vi "DAQNavi Read (Analog 1D DBL 1Chan NSamp).vi"(8 "error in (no error)":errorcluster, 9 "number of samples per channel to read":u32=1000, 10 "timeout":dbl=10.0, 11 "task in":i32) -> (0 "error out":errorcluster, 1 "markBuf":cluster{"Data Index":i64, "SrcId":i64}[](array[cluster]), 2 "data":dbl[](array[numeric]), 3 "task out":i32)   [LabVIEW 2020]
uses:
  DAQNavi_LV.dll
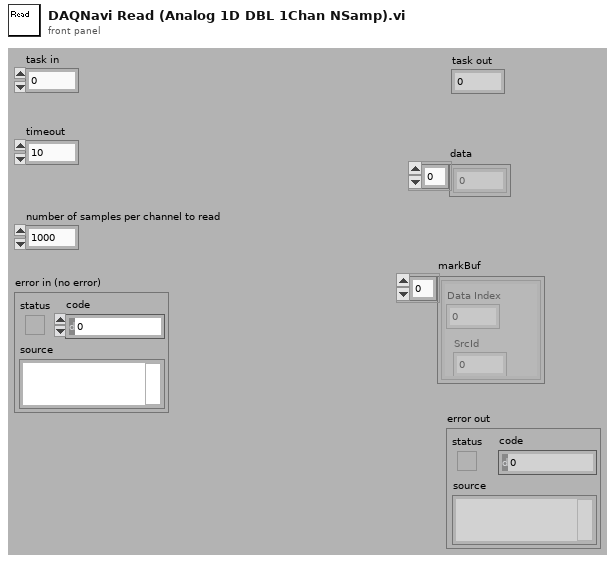
[diagram p1: front panel]
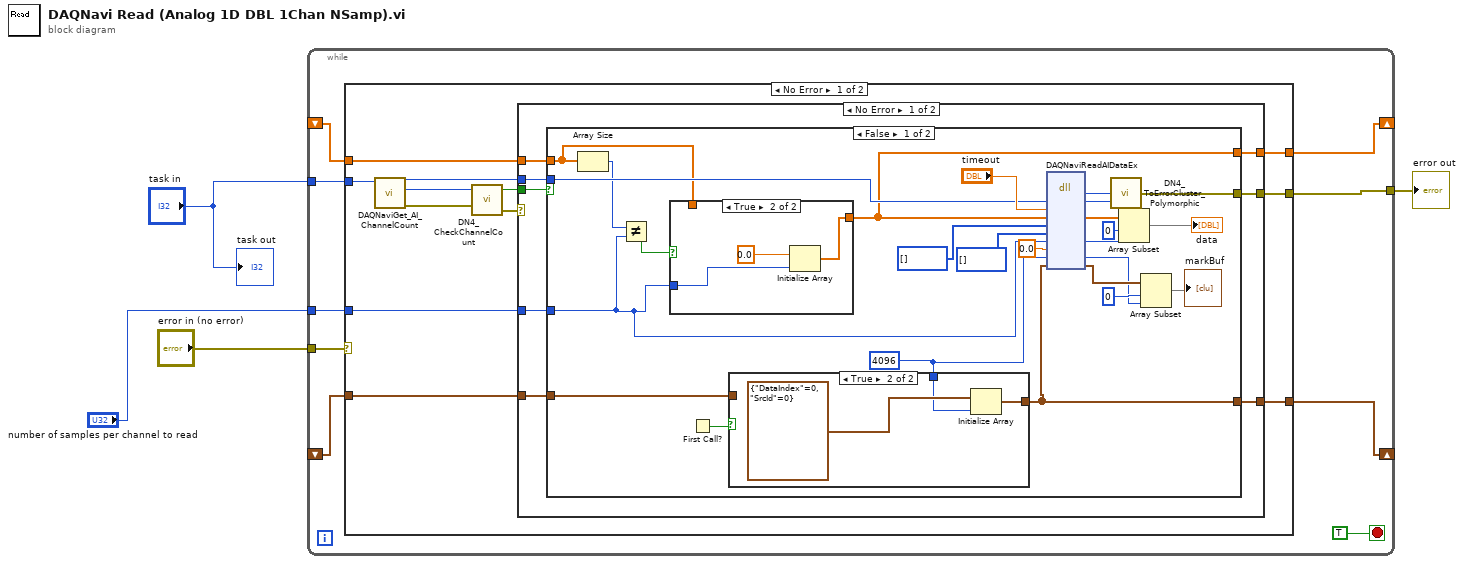
[diagram p0: block diagram]
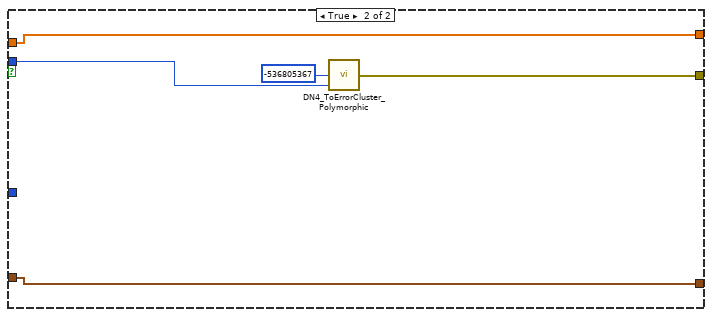
[diagram p4: hidden frame]
diagram:
  n1 = while {
    tunnel: "error in (no error)" -> [w13]
    tunnel: [w12] -> w3
    tunnel: "task in" -> [w11]
    tunnel: "number of samples per channel to read" -> [w10]
    shift-right: [w8] -> _
    shift-left: _ -> [w7]
    shift-right: [w6] -> _
    shift-left: _ -> [w5]
    stop <- TRUE stop-if-true
    n2 = case shown="No Error" w13 {
      selector: w13 -> [_ w77]
      tunnel: w11 -> [w24 _]
      tunnel: [w25 w77] -> w12
      tunnel: w10 -> [w18 _]
      tunnel: [w17 w76] -> w8
      tunnel: w7 -> [w16 w76]
      tunnel: [w15 w75] -> w6
      tunnel: w5 -> [w14 w75]
      frame No Error {
        n3 = call "DAQNaviGet_AI_ChannelCount.vi"("task in"=w24) -> ("error out"=w22:errorcluster, "channel count"=w23:i32, "task out"=w19:i32)  [unwired: 1 in, 7 out]
        n4 = call "DN4_CheckChannelCount.vi"("error out"=w22, "channel count"=w23) -> ("error IO"=w20:errorcluster, "greater than 1?"=w21:bool)  [unwired: 2 out]
        n5 = case shown="No Error" w20 {
          selector: w20 -> [_ w74]
          tunnel: w21 -> [w33 _]
          tunnel: [w32 w74] -> w25
          tunnel: w19 -> [w31 _]
          tunnel: w18 -> [w30 _]
          tunnel: [w29 w73] -> w17
          tunnel: w16 -> [w28 w73]
          tunnel: [w27 w72] -> w15
          tunnel: w14 -> [w26 w72]
          frame No Error {
            n6 = case shown="False" w33 {
              tunnel: [w54 w70] -> w32
              tunnel: w31 -> [w53 w69]
              tunnel: w30 -> [w43 _]
              tunnel: [w45 w68] -> w29
              tunnel: w28 -> [w44 w68]
              tunnel: [w38 w67] -> w27
              tunnel: w26 -> [w40 w67]
              frame False {
                w39 = 4096 ("startTime")
                n7 = Array Size(array=w44) -> (size(s)=w47:i32)
                n8 = Not Equal?(x=w47, y=w43) -> (x != y?=w46:bool)
                n9 = case shown="True" w46 {
                  tunnel: w43 -> [_ w65]
                  tunnel: [w63 w64] -> w45
                  tunnel: w44 -> [w63 _]
                  frame False {
                  }
                  frame True {
                    n10 = Initialize Array(0.0 ("element"), w65) -> (w64:dbl[])
                  }
                }
                n11 = First Call?() -> (First Call?: T/F=w41:bool)
                n12 = case shown="True" w41 {
                  tunnel: w39 -> [_ w61]
                  tunnel: [w59 w60] -> w38
                  tunnel: w40 -> [w59 _]
                  frame False {
                  }
                  frame True {
                    n13 = Initialize Array(cluster{"DataIndex":i64, "SrcId":i64} {"DataIndex"=0, "SrcId"=0}, w61) -> (w60:cluster{"DataIndex":i64, "SrcId":i64}[])
                  }
                }
                n14 = dll-call lib="DAQNavi_LV.dll" fn="DAQNaviReadAIDataEx"("taskID"=w53, "timeout"="timeout", "scaledData"=w45, "rawData16"=u16[] [], "rawData32"=u32[] [], "samples"=w43, "startTime"=0.0, "markCount"=w39, "markBuf"=w38) -> ("return type"=w55:i32, "taskID"=w48:i32, "scaledData"=w52:dbl[], "samples"=w50:u32, "markCount"=w35:i32, "markBuf"=w37:cluster{"DataIndex":i64, "SrcId":i64}[])  [unwired: 4 in, 5 out]
                n15 = call "DN4_ToErrorCluster_Polymorphic.vi"("task id"=w48, "error code"=w55) -> ("error out"=w54:errorcluster)  [unwired: 3 out]
                n16 = Array Subset(array=w52, index=0, length=w50) -> (→"data":dbl[])
                n17 = Array Subset(array=w37, index=0, length=w35) -> (→"markBuf":cluster{"DataIndex":i64, "SrcId":i64}[])
              }
              frame True {
                n18 = call "DN4_ToErrorCluster_Polymorphic.vi"("task id"=w69, "error code"=-536805367 ("error code (0)")) -> ("error out"=w70:errorcluster)  [unwired: 3 out]
              }
            }
          }
          frame Error {
          }
        }
      }
      frame Error {
      }
    }
  }
  "error out" <- w3
  "task out" <- "task in"
